vi "Create Attribute (String).vi"(10 "Value":string, 11 "Name":string) -> (3 "Attribute":refnum<class "Attribute.lvclass">)   [LabVIEW 2020, in "VILab.lvlib" / "Attribute.lvclass"]
uses:
  Attribute.lvclass
  Data Item/Data Item.lvclass/Data Item.ctl
  Attribute.lvclass/Attribute.ctl
  Data Item/Data Item.lvclass
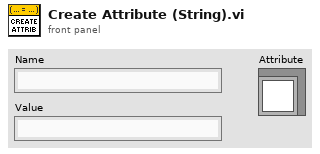
[diagram p1: front panel]
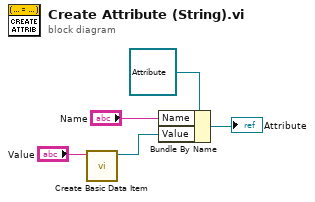
[diagram p0: block diagram]
diagram:
  n1 = call "Create Basic Data Item.vi"("Content"="Value") -> ("New Data Item"=w1:refnum<class "Data Item.lvclass">)  [unwired: 10 in]
  n2 = Bundle By Name(cluster=refnum<class "Attribute.lvclass"> refnum ("VILab.lvlib:Attribute.lvclass"), "Name"="Name", "Value"=w1) -> (→"Attribute":refnum<class "Attribute.lvclass">)
